vi "Warp Perspective.vi"   [LabVIEW 2020, in "image.lvlib"]
doc: "Warp the Source Image based on the 3x3 Warp Matrix.\n\nA Warp Matrix can be computed using the \"Get Perspective Transform.vi\""
uses:
  image.lvlib
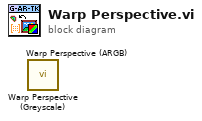
[diagram p0: block diagram]
diagram:
  n1 = call "Warp Perspective (Greyscale).vi"() -> ()  [unwired: 10 in, 2 out]
  n2 = call "Warp Perspective (ARGB).vi"() -> ()  [unwired: 10 in, 2 out]
